vi "Resample Unequally-Sampled Time Series.vi"() -> ()   [LabVIEW 2023]
doc: "This example shows how to convert a unequally-sampled series into an equally-sampled time series with the TSA Resampling VI.\n\n<b>Instructions:</b>\n1) Run this VI.\n2) Set the new sampling rate.\n3) Observe the resampled signal against the original signal."
uses:
  <vilib>/addons/Time Series Analysis/Series Preprocess.llb/TSA Resampling (Unequal).vi
  <vilib>/addons/_Advanced Signal Processing/NI_AdvSigProcTSA.lvlib
panel:
  in  "New sampling rate":dbl=30.0
  out "Resampled Time Series":waveform(dbl)(graph)
  out "Original Time Series":cluster{"time index":dbl[], "time series":dbl[]}(graph)
  in  "stop":bool
  # "Overview: Shows how to convert a unequally-sampled series into an equally-sampled time series with the TSA Resampling VI.\nRequirements: LabVIEW Full Development System, Advanced Signal Processing Toolkit\nInstructions: \n1. Run this VI.\n2. Set the new sampling rate.\n3. Observe the resampled signal against the original signal.\n4.  Click Stop to stop the VI."
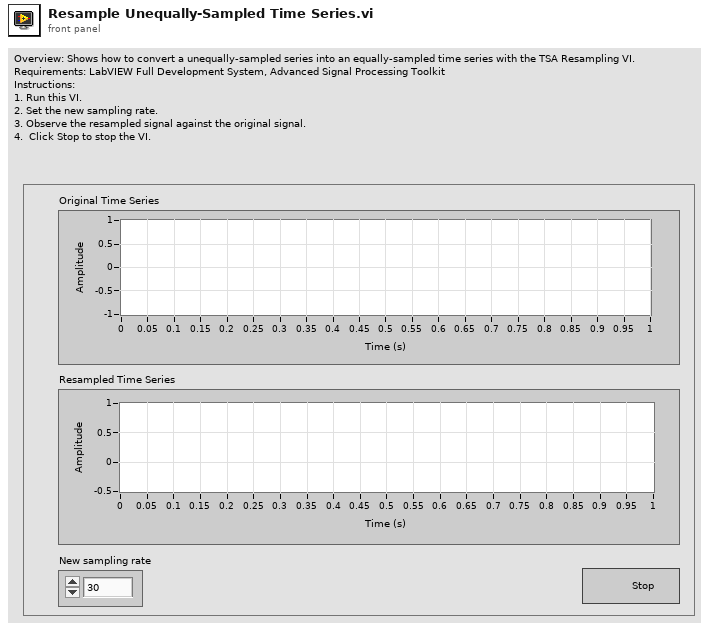
[diagram p1: front panel]
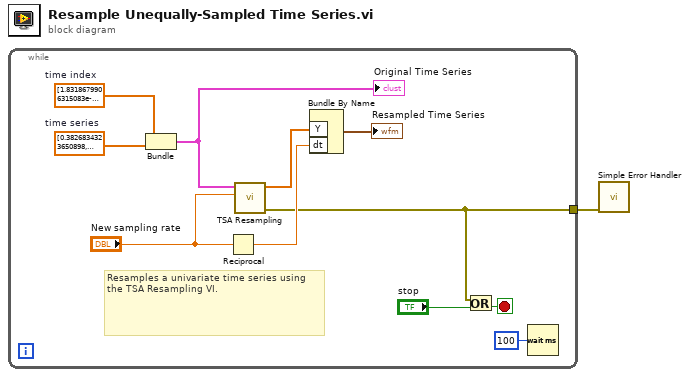
[diagram p0: block diagram]
diagram:
  n1 = while {
    tunnel: [w3] -> w1
    stop <- w11 stop-if-true
    w4 = dbl[] [0.3826834323650898, 0.7071067811865476, 0.9238795325112867, 1.0, 0.9238795325112867, 0.7071067811865475, 0.38268343236508967, -1.0560129160008813e-16, -0.3826834323650899, -0.7071067811865476]  # time series
    w5 = dbl[] [1.8318679906315083e-14, 0.30102999566399946, 0.4771212547196807, 0.6020599913279807, 0.6989700043360371, 0.778151250383662, 0.8450980400142751, 0.903089986991962, 0.9542425094393432, 1.0000000000000184]  # time index
    # "Resamples a univariate time series using the TSA Resampling VI."
    n2 = Bundle("time index"=w5, "time series"=w4) -> (w6:cluster{"time index":dbl[], "time series":dbl[]})  [unwired: 1 out]
    "Original Time Series" <- w6
    n3 = Reciprocal(x="New sampling rate") -> (1/x=w8:dbl)
    n4 = call-poly <vilib>:"TSA Resampling.vi"("new sampling rate"="New sampling rate", "Xt"=w6) -> ("error out"=w3:errorcluster, "Xt resampled"=w10:dbl[])  [unwired: 1 in, 7 out]
    n5 = Bundle By Name("Y"=w10, "dt"=w8) -> (→"Resampled Time Series":waveform(dbl))  [unwired: 1 out]
    n6 = Or(x=w3, y="stop") -> (x .or. y?=w11:bool)
    n7 = Wait (ms)(milliseconds to wait=u32 100) -> ()  [unwired: 1 out]
  }
  n8 = call <vilib>:"Simple Error Handler.vi"("error in (no error)"=w1) -> ()  [unwired: 1 in, 8 out]
